vi "Open.vi"(8 "error in (no error)":errorcluster, 11 "Clock Time in":refnum<class "Clock Time.lvclass">) -> (0 "error out":errorcluster, 3 "Clock Time out":refnum<class "Clock Time.lvclass">)   [LabVIEW 2024, in "Clock Time.lvclass"]
doc: "Clock Time.lvclass:Open.vi\n\nThis VI does no real action but is needed for compatibility with the Bus class.\n\nInstrument Communication Module Version 1.0\nAugust, 2017 Original Code Consulting David Thomson\n www.originalcode.com"
uses:
  Clock Time.lvclass
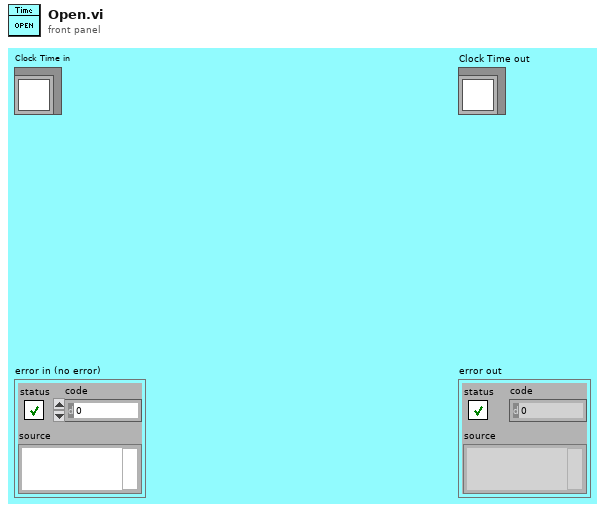
[diagram p1: front panel]
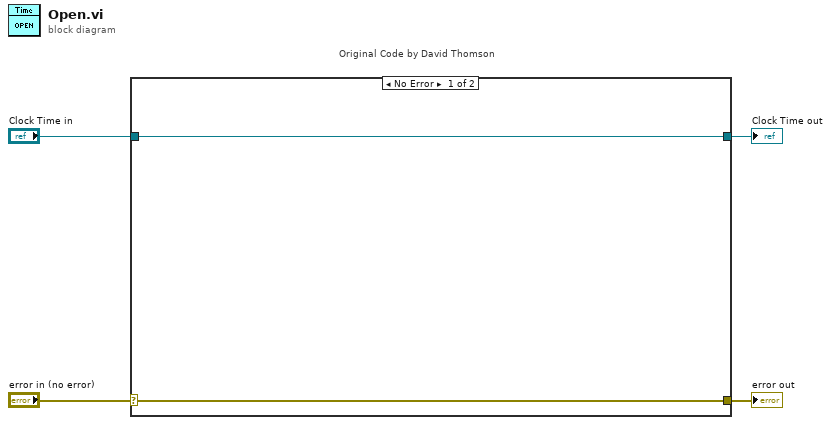
[diagram p0: block diagram]
diagram:
  n1 = case "Original Code by David Thomson" shown="No Error" "error in (no error)" {
    selector: "error in (no error)" -> [w5 w8]
    tunnel: [w5 w8] -> w3
    tunnel: [w6 w7] -> w1
    tunnel: "Clock Time in" -> [w6 w7]
    frame No Error {
    }
    frame Error {
    }
  }
  "error out" <- w3
  "Clock Time out" <- w1
